vi "hour_angle.vi"(1 "Rotation period (hours)":dbl=24.0, 2 "Time (hour of day since midnight)":dbl) -> (0 "Hour angle h (rad)":dbl=3.141592653589793)   [LabVIEW 2012]
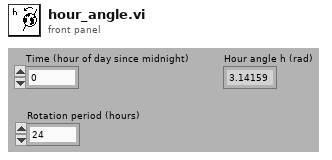
[diagram p1: front panel]
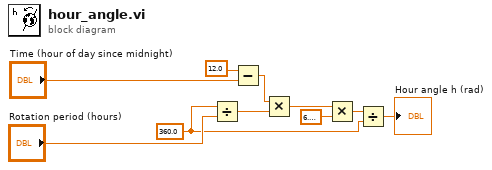
[diagram p0: block diagram]
diagram:
  w2 = 360.0 ("y")
  n1 = Divide(x=w2, y="Rotation period (hours)") -> (x/y=w1:dbl)
  n2 = Subtract(x=12.0, y="Time (hour of day since midnight)") -> (x-y=w6:dbl)
  n3 = Multiply(x=w6, y=w1) -> (x*y=w5:dbl)
  n4 = Multiply(x=w5, y=6.283185307179586) -> (x*y=w9:dbl)
  n5 = Divide(x=w9, y=w2) -> (x/y=→"Hour angle h (rad)":dbl)
